vi "Get Keywords.vi"(8 "error in (no error)":errorcluster, 11 "Structure If Else in":refnum<class "Structure If Else.lvclass">) -> (0 "error out":errorcluster, 2 "Keywords":string[](array[string]), 3 "Structure If Else out":refnum<class "Structure If Else.lvclass">)   [LabVIEW 2019, in "Structure If Else.lvclass"]
uses:
  Structure If Else.lvclass
  functionsbase/functionbase.lvclass
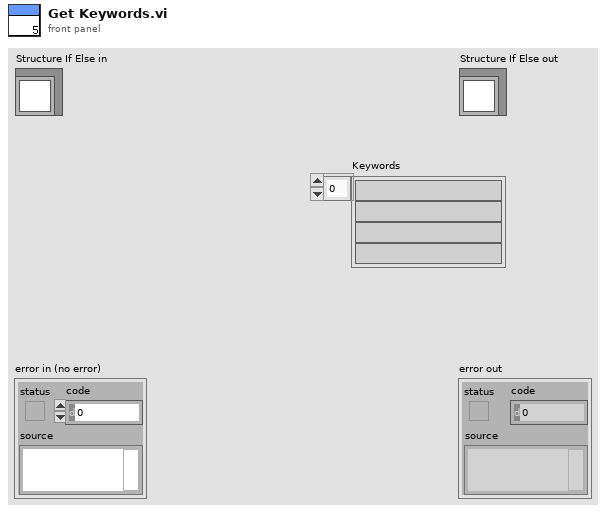
[diagram p1: front panel]
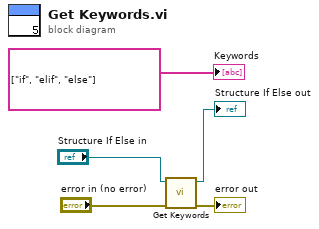
[diagram p0: block diagram]
diagram:
  n1 = call-parent "Get Keywords.vi"("error in (no error)"="error in (no error)", "functionbase in"="Structure If Else in") -> ("error out"=→"error out":errorcluster, "functionbase out"=→"Structure If Else out":refnum<class "Structure If Else.lvclass">)  [unwired: 7 in, 1 out]
  "Keywords" <- string[] ["if", "elif", "else"] ("Keywords")
